vi "Encode URICompmnent.vi"(1 "URI":string) -> (0 "encodeURIComponent":string)   [LabVIEW 2017, in "Encode Base64.lvlib"]
uses:
  Encode Base64.lvlib
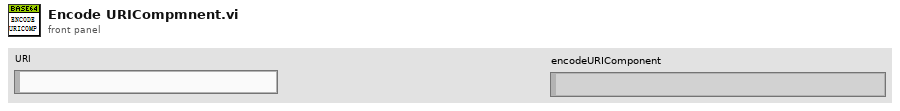
[diagram p1: front panel]
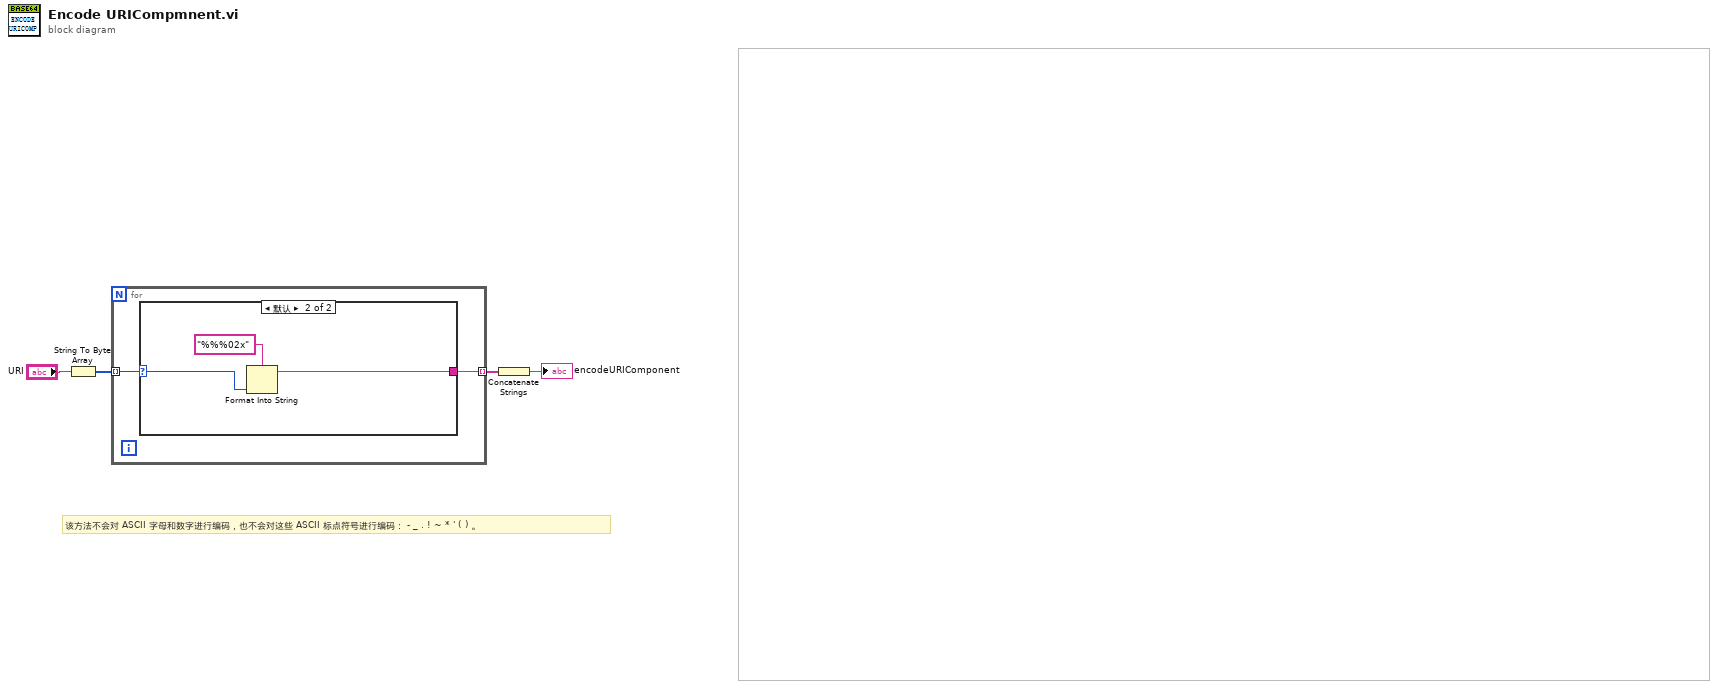
[diagram p0: block diagram]
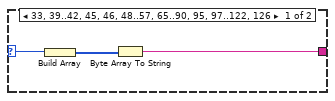
[diagram p2: hidden frame]
diagram:
  # "该方法不会对 ASCII 字母和数字进行编码，也不会对这些 ASCII 标点符号进行编码： - _ . ! ~ * ' ( ) 。"
  n1 = String To Byte Array(string="URI") -> (unsigned byte array=w3:u8[])
  n2 = for {
    tunnel: w3 -> [w6] mode=indexing
    tunnel: [w5] -> w2 mode=indexing
    n3 = case shown="默认" w6 {
      selector: w6 -> [w9 w10]
      tunnel: [w7 w11] -> w5
      frame 33, 39..42, 45, 46, 48..57, 65..90, 95, 97..122, 126 {
        n4 = Build Array(w9) -> (w8:u8[])
        n5 = Byte Array To String(unsigned byte array=w8) -> (string=w7:string)
      }
      frame Default {
        n6 = Format Into String(format string="%%%02x", w10) -> (resulting string=w11:string)  [unwired: 2 in, 1 out]
      }
    }
  }
  n7 = Concatenate Strings(w2) -> (→"encodeURIComponent":string)
